vi "scan RP100 voltage.vi"(7 "data":refnum<queue>, 8 "error in (no error)":errorcluster, 11 "config in":T8={"initialize"=enum."SR830", "6221"={"6221 Resource"="GPIB1::10::INSTR", "Delta status"=FALSE, "电流|RMS(A)"=0.0}, "SR830+6221"={"source"=0, "Current(A)"=0.0, "阻抗(Ohm)"=0.0, "SR830 1"=FALSE, "SR830 2"=FALSE, "SR830 3"=FALSE, "SR830 4"=FALSE, "VISA 1"="GPIB1::1::INSTR", "VISA 2"="GPIB1::2::INSTR", "VISA 3"="GPIB1::3::INSTR", "VISA 4"="GPIB1::4::INSTR", "Reserve 1"=-1, "Reserve 2"=-1, "Reserve 3"=-1, "Reserve 4"=-1, "Sensitivity 1"=-1, "Sensitivity 2"=0, "Sensitivity 3"=-1, "Sensitivity 4"=-1, "量程入 1"=0, "量程入 2"=0, "量程入 3"=0, "量程入 4"=0}, "2400"={"2400"=FALSE, "VISA"="GPIB0::9::INSTR", "Output Level (0)"=1e-05, "Compliance  Level (0.1)"=10.0, "2400ch\n\n2400ch"=[]}, "ch"={"ch"=[], "current"=[], "change?"=[], "holding current\nwhen change ch?"=TRUE}, "Instrument"={"limit"={"Field limit"=0.0, "Field rate limit"=0.0, "Temp limit"=0.0, "Temp low limit"=0.0, "Temp rate limit "=0.0}, "genarl"={"行数"=refnum, "编辑列表框？"=refnum, "列表框"=refnum, "camg 振荡状态"=refnum, "Aborting"=refnum, "数据文件"=refnum, "warning"=refnum, "vi路径"="", "Instrument Type"=enum."PPMS"}, "cmag"={"TM620"="COM3", "M24C Resource"="GPIB0::1::INSTR", "4G supply"="GPIB0::13::INSTR", "Temp Status 24C"=refnum, "Temp"=refnum, "9T信号"=refnum, "4g supply status"=refnum, "in-plane"="", "out-plane"="", "in-plane signal"=FALSE, "out-plane signal"=FALSE, "in plane 信号"=refnum, "pzt volt"=refnum, "camg Rate"=refnum}, "lengtou2"={"750 visa"="", "750 rotate"="", "semaphore 340"=refnum, "semaphore 750"=refnum, "750 field status"=refnum, "Input (0:A) 340"=0, "340 Resource"="GPIB0::14::INSTR", "340 Status"=refnum, "Input (0:B) 340"=0, "Loop (0: 1)"=1, "Loop (1: 1)"=0, "TCP master instance"=refnum}, "lengtou"={"TCP master instance"=refnum, "335 Status"=refnum, "335 Resource "="GPIB0::24::INSTR", "Input (0:A) 335"=0, "Input (0:B) 335"=1, "Heater Output (1:1) 335"=1, "semaphore 335"=refnum}, "325 for test"={"quantum design"=refnum, "semaphore 325"=refnum, "325 Resource "="GPIB0::13::INSTR", "Input (0:A) 325"=0, "Heater Output (1:1) 325"=1, "325 Status"=refnum}}, "Aborting"=refnum, "数据文件"=refnum, "warning"=refnum, "2614B"={"2614B chA"=FALSE, "2614B chB"=FALSE, "VISA"="GPIB1::5::INSTR"}, "33522b"={"33522b resource name"="GPIB0::16::INSTR", "零电压"=0.0, "最大电压"=150.0, "间隔"=3.0, "最小电压"=-50.0, "开始扫温？"=FALSE, "loop"=3}, "gating type"=enum."2614(daul)", "RP100"={"RP100 VISA"="", "Slew"=0.0, "Voltage1"=0.0, "Reset?"=FALSE, "Voltage 2"=0.0, "interval"=0.0, "scan temp?"=FALSE}, "E4980AL"={"E4980AL VISA"="", "Function (0: Cp-D)"=0, "Signal Frequency (1000 Hz)"=1000.0}} {"E4980AL"."Function (0: Cp-D)" items=["Cp-D", "Cp-Q", "Cp-G", "Cp-Rp", "Cs-D", "Cs-Q", "Cs-Rs", "Lp-D", "Lp-Q", "Lp-G", "Lp-Rp", "Lp-Rdc", "Ls-D", "Ls-Q", "Ls-Rs", "Ls-Rdc", "R-X", "Z-thd", "Z-thr", "G-B", "Y-thd", "Y-thr", "Vdc-Idc"]; "33522b"."loop" items=["0", "1", "2", "3"]; "Instrument"."325 for test"."Heater Output (1:1) 325" items=["1"=1, "2"=2]; "Instrument"."325 for test"."Input (0:A) 325" items=["A", "B"]; "Instrument"."lengtou"."Heater Output (1:1) 335" items=["1"=1, "2"=2]; "Instrument"."lengtou"."Input (0:B) 335" items=["A", "B"]; "Instrument"."lengtou"."Input (0:A) 335" items=["A", "B"]; "Instrument"."lengtou2"."Loop (1: 1)" items=["1", "2"]; "Instrument"."lengtou2"."Loop (0: 1)" items=["1", "2"]; "Instrument"."lengtou2"."Input (0:B) 340" items=["A", "B", "C", "D"]; "Instrument"."lengtou2"."Input (0:A) 340" items=["A", "B", "C", "D"]; "SR830+6221"."Sensitivity 4" items=["Auto Gain"=-1, "2 nV/fA"=0, "5 nV/fA"=1, "10 nV/fA"=2, "20 nV/fA"=3, "50 nV/fA"=4, "100 nV/fA"=5, "200 nV/fA"=6, "500 nV/fA"=7, "1 uV/pA"=8, "2 uV/pA"=9, "5 uV/pA"=10, "10 uV/pA"=11, "20 uV/pA"=12, "50 uV/pA"=13, "100 uV/pA"=14, "200 uV/pA"=15, "500 uV/pA"=16, "1 mV/nA"=17, "2 mV/nA"=18, "5 mV/nA"=19, "10 mV/nA"=20, "20 mV/nA"=21, "50 mV/nA"=22, "100 mV/nA"=23, "200 mV/nA"=24, "500 mV/mA"=25, "1 V/uA"=26]; "SR830+6221"."Sensitivity 3" items=["Auto Gain"=-1, "2 nV/fA"=0, "5 nV/fA"=1, "10 nV/fA"=2, "20 nV/fA"=3, "50 nV/fA"=4, "100 nV/fA"=5, "200 nV/fA"=6, "500 nV/fA"=7, "1 uV/pA"=8, "2 uV/pA"=9, "5 uV/pA"=10, "10 uV/pA"=11, "20 uV/pA"=12, "50 uV/pA"=13, "100 uV/pA"=14, "200 uV/pA"=15, "500 uV/pA"=16, "1 mV/nA"=17, "2 mV/nA"=18, "5 mV/nA"=19, "10 mV/nA"=20, "20 mV/nA"=21, "50 mV/nA"=22, "100 mV/nA"=23, "200 mV/nA"=24, "500 mV/mA"=25, "1 V/uA"=26]; "SR830+6221"."Sensitivity 1" items=["Auto Gain"=-1, "2 nV/fA"=0, "5 nV/fA"=1, "10 nV/fA"=2, "20 nV/fA"=3, "50 nV/fA"=4, "100 nV/fA"=5, "200 nV/fA"=6, "500 nV/fA"=7, "1 uV/pA"=8, "2 uV/pA"=9, "5 uV/pA"=10, "10 uV/pA"=11, "20 uV/pA"=12, "50 uV/pA"=13, "100 uV/pA"=14, "200 uV/pA"=15, "500 uV/pA"=16, "1 mV/nA"=17, "2 mV/nA"=18, "5 mV/nA"=19, "10 mV/nA"=20, "20 mV/nA"=21, "50 mV/nA"=22, "100 mV/nA"=23, "200 mV/nA"=24, "500 mV/mA"=25, "1 V/uA"=26]; "SR830+6221"."Sensitivity 2" items=["Auto Gain"=-1, "2 nV/fA"=0, "5 nV/fA"=1, "10 nV/fA"=2, "20 nV/fA"=3, "50 nV/fA"=4, "100 nV/fA"=5, "200 nV/fA"=6, "500 nV/fA"=7, "1 uV/pA"=8, "2 uV/pA"=9, "5 uV/pA"=10, "10 uV/pA"=11, "20 uV/pA"=12, "50 uV/pA"=13, "100 uV/pA"=14, "200 uV/pA"=15, "500 uV/pA"=16, "1 mV/nA"=17, "2 mV/nA"=18, "5 mV/nA"=19, "10 mV/nA"=20, "20 mV/nA"=21, "50 mV/nA"=22, "100 mV/nA"=23, "200 mV/nA"=24, "500 mV/mA"=25, "1 V/uA"=26]; "SR830+6221"."Reserve 4" items=["Auto Reserve"=-1, "High Reserve"=0, "Normal"=1, "Low Noise"=2]; "SR830+6221"."Reserve 3" items=["Auto Reserve"=-1, "High Reserve"=0, "Normal"=1, "Low Noise"=2]; "SR830+6221"."Reserve 2" items=["Auto Reserve"=-1, "High Reserve"=0, "Normal"=1, "Low Noise"=2]; "SR830+6221"."Reserve 1" items=["Auto Reserve"=-1, "High Reserve"=0, "Normal"=1, "Low Noise"=2]; "SR830+6221"."source" items=["SR830 1", "SR830 2", "SR830 3", "SR830 4"]}) -> (0 "error out":errorcluster, 3 "config in 2":T1={"initialize"=enum."SR830", "6221"={"6221 Resource"="GPIB0::24::INSTR", "Delta status"=FALSE, "电流|RMS(A)"=0.0}, "SR830+6221"={"source"=0, "Current(A)"=0.0, "阻抗(Ohm)"=0.0, "SR830 1"=FALSE, "SR830 2"=FALSE, "SR830 3"=FALSE, "SR830 4"=FALSE, "VISA 1"="", "VISA 2"="", "VISA 3"="", "VISA 4"="", "Reserve 1"=-1, "Reserve 2"=-1, "Reserve 3"=-1, "Reserve 4"=-1, "Sensitivity 1"=-1, "Sensitivity 2"=-1, "Sensitivity 3"=-1, "Sensitivity 4"=-1, "量程入 1"=0, "量程入 2"=0, "量程入 3"=0, "量程入 4"=0}, "2400"={"2400"=FALSE, "VISA"="GPIB0::9::INSTR", "Output Level (0)"=1e-05, "Compliance  Level (0.1)"=10.0, "ch"=[]}, "ch"={"ch"=[], "current"=[], "change?"=[], "holding current\nwhen change ch?"=FALSE, "current offset"=[]}, "Instrument"={"limit"={"Field limit"=0.0, "Field rate limit"=0.0, "Temp limit"=0.0, "Temp low limit"=0.0, "Temp rate limit "=0.0}, "genarl"={"行数"=refnum, "编辑列表框？"=refnum, "列表框"=refnum, "camg 振荡状态"=refnum, "Aborting"=refnum, "数据文件"=refnum, "warning"=refnum, "vi路径"="", "Instrument Type"=enum."SVSM"}, "cmag"={"TM620"="GPIB0::24::INSTR", "M24C Resource"="GPIB0::24::INSTR", "4G supply"="GPIB0::24::INSTR", "Temp Status 24C"=refnum, "Temp"=refnum, "9T信号"=refnum, "4g supply status"=refnum, "in-plane"="", "out-plane"="", "in-plane signal"=TRUE, "out-plane signal"=FALSE, "in plane 信号"=refnum, "pzt volt"=refnum, "camg Rate"=refnum}, "lengtou2"={"750 visa"="", "750 rotate"="", "semaphore 340"=refnum, "semaphore 750"=refnum, "750 field status"=refnum, "Input (0:A) 340"=1, "340 Resource"="GPIB0::14::INSTR", "340 Status"=refnum, "Input (0:B) 340"=0, "Loop (0: 1)"=1, "Loop (1: 1)"=0, "TCP master instance"=refnum}, "lengtou"={"TCP master instance"=refnum, "335 Status"=refnum, "335 Resource "="GPIB0::24::INSTR", "Input (0:A) 335"=0, "Input (0:B) 335"=0, "Heater Output (1:1) 335"=0, "semaphore 335"=refnum}, "325 for test"={"quantum design"=refnum, "semaphore 325"=refnum, "325 Resource "="GPIB0::13::INSTR", "Input (0:A) 325"=1000, "Heater Output (1:1) 325"=1, "325 Status"=refnum}}, "2614B"={"2614B chA"=FALSE, "2614B chB"=FALSE, "VISA"=""}, "33522b"={"33522b resource name"="GPIB0::16::INSTR", "零电压"=0.0, "最大电压"=148.0, "间隔"=4.0, "最小电压"=-48.0, "loop"=3.0, "压电陶瓷电压(Vpp)"=0.0}, "gating type"=enum."2614(daul)", "层数"=0, "行数"=0, "是否处理"=[], "current 2"=[], "StrainCell"={"RP100 resource name"="GPIB0::16::INSTR", "E4980 resource name"="GPIB0::16::INSTR", "RP100 Reset ?(True)"=TRUE, "Voltage1(V)"=0.0, "Voltage2(V)"=0.0, "interval"=4.0, "slew(V/s)"=1.0}} {"Instrument"."325 for test"."Heater Output (1:1) 325" items=["1"=1, "2"=2]; "Instrument"."325 for test"."Input (0:A) 325" items=["A", "B"]; "Instrument"."lengtou"."Heater Output (1:1) 335" items=["1"=1, "2"=2]; "Instrument"."lengtou"."Input (0:B) 335" items=["A", "B"]; "Instrument"."lengtou"."Input (0:A) 335" items=["A", "B"]; "Instrument"."lengtou2"."Loop (1: 1)" items=["1", "2"]; "Instrument"."lengtou2"."Loop (0: 1)" items=["1", "2"]; "Instrument"."lengtou2"."Input (0:B) 340" items=["A", "B", "C", "D"]; "Instrument"."lengtou2"."Input (0:A) 340" items=["A", "B", "C", "D"]; "SR830+6221"."Sensitivity 4" items=["Auto Gain"=-1, "2 nV/fA"=0, "5 nV/fA"=1, "10 nV/fA"=2, "20 nV/fA"=3, "50 nV/fA"=4, "100 nV/fA"=5, "200 nV/fA"=6, "500 nV/fA"=7, "1 uV/pA"=8, "2 uV/pA"=9, "5 uV/pA"=10, "10 uV/pA"=11, "20 uV/pA"=12, "50 uV/pA"=13, "100 uV/pA"=14, "200 uV/pA"=15, "500 uV/pA"=16, "1 mV/nA"=17, "2 mV/nA"=18, "5 mV/nA"=19, "10 mV/nA"=20, "20 mV/nA"=21, "50 mV/nA"=22, "100 mV/nA"=23, "200 mV/nA"=24, "500 mV/mA"=25, "1 V/uA"=26]; "SR830+6221"."Sensitivity 3" items=["Auto Gain"=-1, "2 nV/fA"=0, "5 nV/fA"=1, "10 nV/fA"=2, "20 nV/fA"=3, "50 nV/fA"=4, "100 nV/fA"=5, "200 nV/fA"=6, "500 nV/fA"=7, "1 uV/pA"=8, "2 uV/pA"=9, "5 uV/pA"=10, "10 uV/pA"=11, "20 uV/pA"=12, "50 uV/pA"=13, "100 uV/pA"=14, "200 uV/pA"=15, "500 uV/pA"=16, "1 mV/nA"=17, "2 mV/nA"=18, "5 mV/nA"=19, "10 mV/nA"=20, "20 mV/nA"=21, "50 mV/nA"=22, "100 mV/nA"=23, "200 mV/nA"=24, "500 mV/mA"=25, "1 V/uA"=26]; "SR830+6221"."Sensitivity 1" items=["Auto Gain"=-1, "2 nV/fA"=0, "5 nV/fA"=1, "10 nV/fA"=2, "20 nV/fA"=3, "50 nV/fA"=4, "100 nV/fA"=5, "200 nV/fA"=6, "500 nV/fA"=7, "1 uV/pA"=8, "2 uV/pA"=9, "5 uV/pA"=10, "10 uV/pA"=11, "20 uV/pA"=12, "50 uV/pA"=13, "100 uV/pA"=14, "200 uV/pA"=15, "500 uV/pA"=16, "1 mV/nA"=17, "2 mV/nA"=18, "5 mV/nA"=19, "10 mV/nA"=20, "20 mV/nA"=21, "50 mV/nA"=22, "100 mV/nA"=23, "200 mV/nA"=24, "500 mV/mA"=25, "1 V/uA"=26]; "SR830+6221"."Sensitivity 2" items=["Auto Gain"=-1, "2 nV/fA"=0, "5 nV/fA"=1, "10 nV/fA"=2, "20 nV/fA"=3, "50 nV/fA"=4, "100 nV/fA"=5, "200 nV/fA"=6, "500 nV/fA"=7, "1 uV/pA"=8, "2 uV/pA"=9, "5 uV/pA"=10, "10 uV/pA"=11, "20 uV/pA"=12, "50 uV/pA"=13, "100 uV/pA"=14, "200 uV/pA"=15, "500 uV/pA"=16, "1 mV/nA"=17, "2 mV/nA"=18, "5 mV/nA"=19, "10 mV/nA"=20, "20 mV/nA"=21, "50 mV/nA"=22, "100 mV/nA"=23, "200 mV/nA"=24, "500 mV/mA"=25, "1 V/uA"=26]; "SR830+6221"."Reserve 4" items=["Auto Reserve"=-1, "High Reserve"=0, "Normal"=1, "Low Noise"=2]; "SR830+6221"."Reserve 3" items=["Auto Reserve"=-1, "High Reserve"=0, "Normal"=1, "Low Noise"=2]; "SR830+6221"."Reserve 2" items=["Auto Reserve"=-1, "High Reserve"=0, "Normal"=1, "Low Noise"=2]; "SR830+6221"."Reserve 1" items=["Auto Reserve"=-1, "High Reserve"=0, "Normal"=1, "Low Noise"=2]; "SR830+6221"."source" items=["SR830 1", "SR830 2", "SR830 3", "SR830 4"]})   [LabVIEW 2019]
uses:
  lib/RP100/RP100.lvlib
  nematic/Copy of StrainCell.lvlib
  <vilib>/NI/Modbus Library/API/Master/Modbus Master.lvclass
  C:/Program Files (x86)/National Instruments/LabVIEW 2019/vi.lib/NI/Modbus Library/API/Modbus API.lvclass
  ctl/initialize.ctl
  ctl/Instrument Type.ctl
  ctl/335 state.ctl
  ctl/limit.ctl
  ctl/9T mag field stauts.ctl
  ctl/Instrument.ctl
  ctl/warning.ctl
  ctl/Gating type.ctl
  ctl/config.ctl
  C:/Users/fuyang/Desktop/postdoctor/labview/labview-measure/lib/QDInstrument.dll
  lib/QDInstrument.dll
  jigui/Desktop/labview-measure-master240417/labview-measure-master-230926/configs/Control 1.ctl
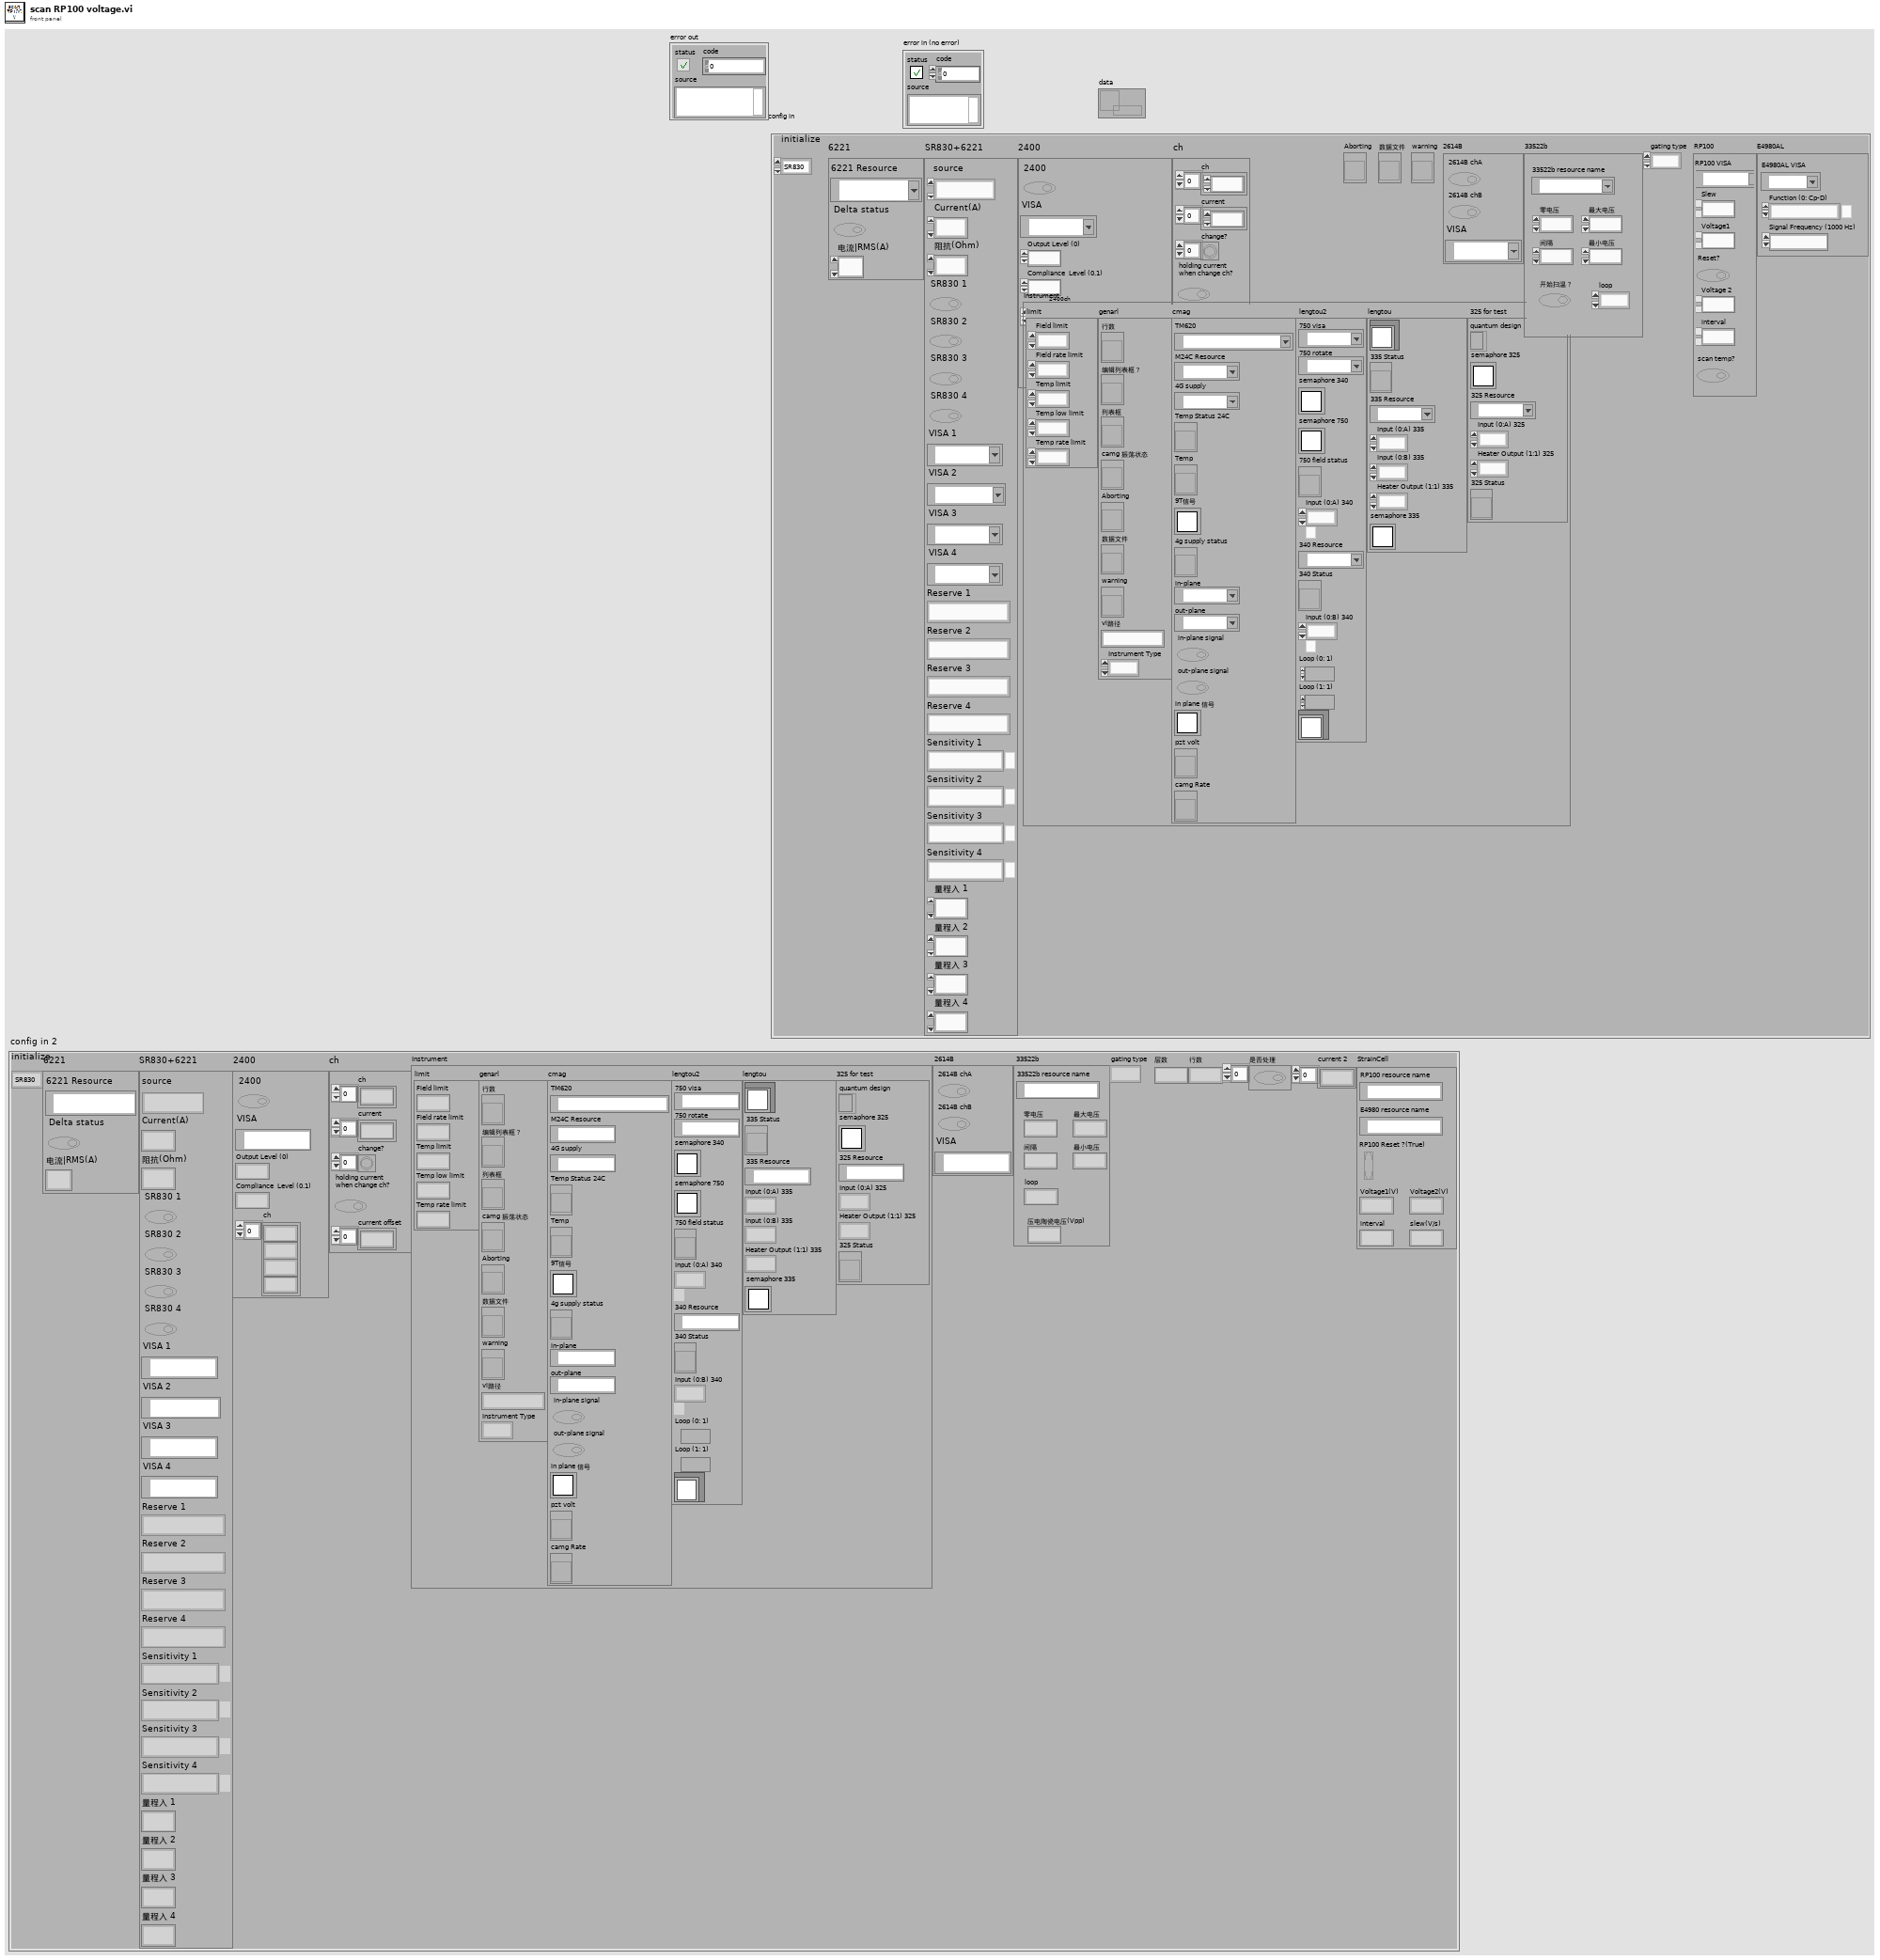
[diagram p1: front panel]
types:
  T1 = typedef "config.ctl" = cluster{"initialize":T2, "6221":cluster{"6221 Resource":refnum<visa-resource-name>, "Delta status":bool, "电流|RMS(A)":dbl}, "SR830+6221":cluster{"source":u16, "Current(A)":dbl, "阻抗(Ohm)":dbl, "SR830 1":bool, "SR830 2":bool, "SR830 3":bool, "SR830 4":bool, "VISA 1":refnum<visa-resource-name>, "VISA 2":refnum<visa-resource-name>, "VISA 3":refnum<visa-resource-name>, "VISA 4":refnum<visa-resource-name>, "Reserve 1":i16, "Reserve 2":i16, "Reserve 3":i16, "Reserve 4":i16, "Sensitivity 1":i16, "Sensitivity 2":i16, "Sensitivity 3":i16, "Sensitivity 4":i16, "量程入 1":i32, "量程入 2":i32, "量程入 3":i32, "量程入 4":i32}, "2400":cluster{"2400":bool, "VISA":refnum<visa-resource-name>, "Output Level (0)":dbl, "Compliance  Level (0.1)":dbl, "ch":i32[]}, "ch":cluster{"ch":i32[], "current":dbl[], "change?":bool[], "holding current\nwhen change ch?":bool, "current offset":dbl[]}, "Instrument":T3, "2614B":cluster{"2614B chA":bool, "2614B chB":bool, "VISA":refnum<visa-resource-name>}, "33522b":cluster{"33522b resource name":refnum<visa-resource-name>, "零电压":dbl, "最大电压":dbl, "间隔":dbl, "最小电压":dbl, "loop":dbl, "压电陶瓷电压(Vpp)":dbl}, "gating type":T7, "层数":i32, "行数":i32, "是否处理":bool[], "current 2":dbl[], "StrainCell":cluster{"RP100 resource name":refnum<visa-resource-name>, "E4980 resource name":refnum<visa-resource-name>, "RP100 Reset ?(True)":bool, "Voltage1(V)":dbl, "Voltage2(V)":dbl, "interval":dbl, "slew(V/s)":dbl}}
  T2 = typedef "initialize.ctl" = enum16{"SR830", "keithley6221-SR830", "Delta", "Delta-tunnelling", "keithley6221-2182-DC", "PZT", "StrainCell", "4200"}
  T3 = typedef "Instrument.ctl" = cluster{"limit":T4, "genarl":cluster{"行数":refnum<vi>, "编辑列表框？":refnum<vi>, "列表框":refnum<vi>, "camg 振荡状态":refnum<vi>, "Aborting":refnum<vi>, "数据文件":refnum<vi>, "warning":refnum<vi>, "vi路径":string, "Instrument Type":T5}, "cmag":cluster{"TM620":refnum<visa-resource-name>, "M24C Resource":refnum<visa-resource-name>, "4G supply":refnum<visa-resource-name>, "Temp Status 24C":refnum<vi>, "Temp":refnum<vi>, "9T信号":T6, "4g supply status":refnum<vi>, "in-plane":refnum<visa-resource-name>, "out-plane":refnum<visa-resource-name>, "in-plane signal":bool, "out-plane signal":bool, "in plane 信号":T6, "pzt volt":refnum<vi>, "camg Rate":refnum<vi>}, "lengtou2":cluster{"750 visa":refnum<visa-resource-name>, "750 rotate":refnum<visa-resource-name>, "semaphore 340":T6, "semaphore 750":T6, "750 field status":refnum<vi>, "Input (0:A) 340":u16, "340 Resource":refnum<visa-resource-name>, "340 Status":refnum<vi>, "Input (0:B) 340":u16, "Loop (0: 1)":u16, "Loop (1: 1)":u16, "TCP master instance":refnum<class "Modbus Master.lvclass">}, "lengtou":cluster{"TCP master instance":refnum<class "Modbus Master.lvclass">, "335 Status":refnum<vi>, "335 Resource ":refnum<visa-resource-name>, "Input (0:A) 335":u16, "Input (0:B) 335":u16, "Heater Output (1:1) 335":u16, "semaphore 335":T6}, "325 for test":cluster{"quantum design":refnum<k24>, "semaphore 325":T6, "325 Resource ":refnum<visa-resource-name>, "Input (0:A) 325":u16, "Heater Output (1:1) 325":u16, "325 Status":refnum<vi>}}
  T4 = typedef "limit.ctl" = cluster{"Field limit":dbl, "Field rate limit":dbl, "Temp limit":dbl, "Temp low limit":dbl, "Temp rate limit ":dbl}
  T5 = typedef "Instrument Type.ctl" = enum16{"PPMS", "VersaLab", "DynaCool", "SVSM", "PPMS-Rotate", "Lakeshore335", "2T cmag", "9T mag old", "9T cmag", "9T cmag DAC", "9T cmag rotate", "test"}
  T6 = typedef "Semaphore RefNum" = refnum<k1>
  T7 = typedef "Gating type.ctl" = enum32{"null", "2614(daul)", "2400", "6517B"}
  T8 = typedef "config.ctl" = cluster{"initialize":T2, "6221":cluster{"6221 Resource":refnum<visa-resource-name>, "Delta status":bool, "电流|RMS(A)":dbl}, "SR830+6221":cluster{"source":u16, "Current(A)":dbl, "阻抗(Ohm)":dbl, "SR830 1":bool, "SR830 2":bool, "SR830 3":bool, "SR830 4":bool, "VISA 1":refnum<visa-resource-name>, "VISA 2":refnum<visa-resource-name>, "VISA 3":refnum<visa-resource-name>, "VISA 4":refnum<visa-resource-name>, "Reserve 1":i16, "Reserve 2":i16, "Reserve 3":i16, "Reserve 4":i16, "Sensitivity 1":i16, "Sensitivity 2":i16, "Sensitivity 3":i16, "Sensitivity 4":i16, "量程入 1":i32, "量程入 2":i32, "量程入 3":i32, "量程入 4":i32}, "2400":cluster{"2400":bool, "VISA":refnum<visa-resource-name>, "Output Level (0)":dbl, "Compliance  Level (0.1)":dbl, "2400ch\n\n2400ch":T9[]}, "ch":cluster{"ch":i32[], "current":dbl[], "change?":bool[], "holding current\nwhen change ch?":bool}, "Instrument":T3, "Aborting":refnum<vi>, "数据文件":refnum<vi>, "warning":refnum<vi>, "2614B":cluster{"2614B chA":bool, "2614B chB":bool, "VISA":refnum<visa-resource-name>}, "33522b":cluster{"33522b resource name":refnum<visa-resource-name>, "零电压":dbl, "最大电压":dbl, "间隔":dbl, "最小电压":dbl, "开始扫温？":bool, "loop":u16}, "gating type":T7, "RP100":cluster{"RP100 VISA":refnum<visa-resource-name>, "Slew":dbl, "Voltage1":dbl, "Reset?":bool, "Voltage 2":dbl, "interval":dbl, "scan temp?":bool}, "E4980AL":cluster{"E4980AL VISA":refnum<visa-resource-name>, "Function (0: Cp-D)":u16, "Signal Frequency (1000 Hz)":dbl}}
  T9 = typedef "Control 1.ctl" = i32
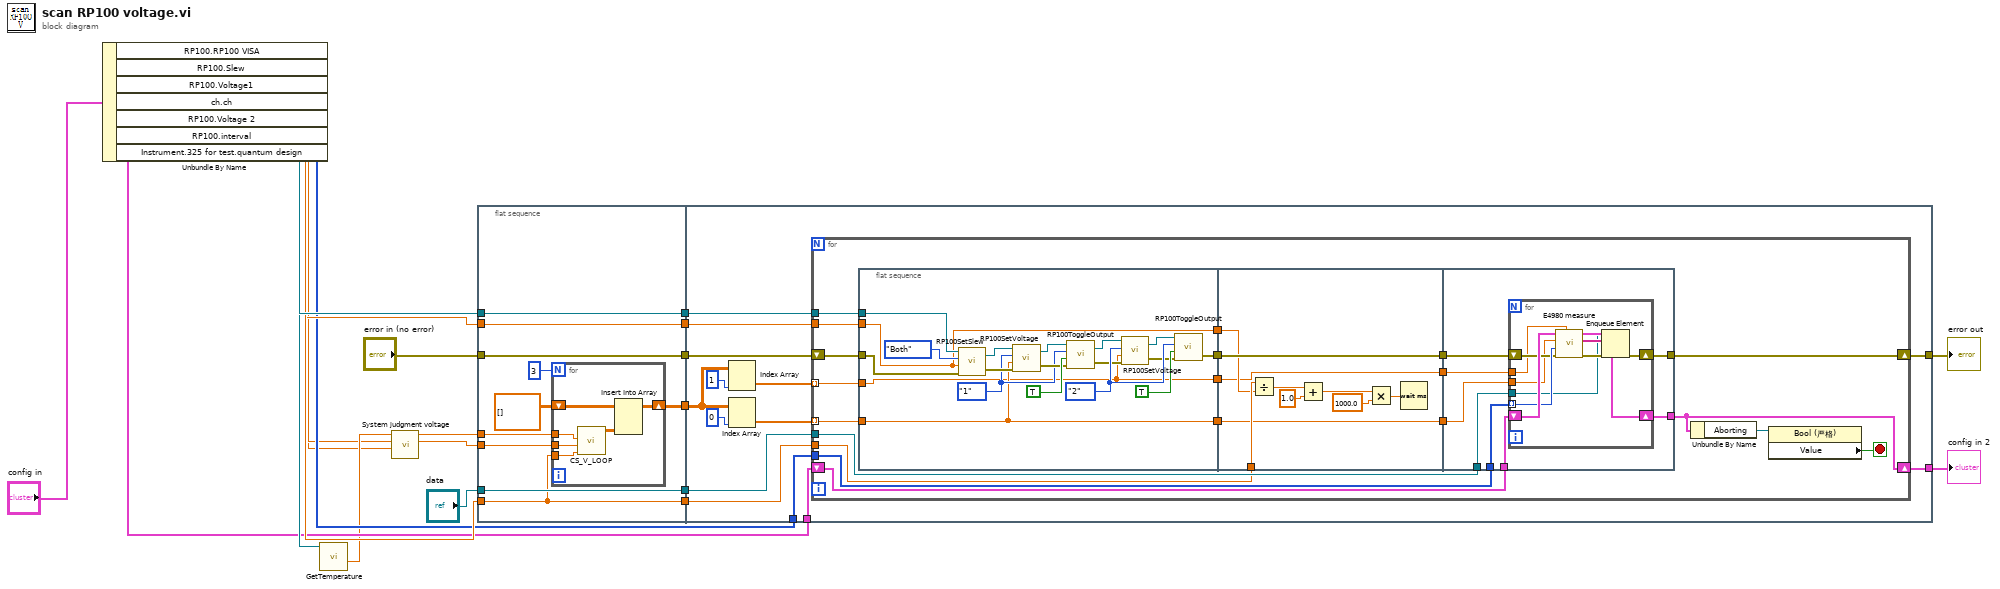
[diagram p0: block diagram]
diagram:
  n1 = Unbundle By Name("config in") -> ("RP100.RP100 VISA"=w19:refnum<visa-resource-name>, "RP100.Slew"=w12:dbl, "RP100.Voltage1"=w4:dbl, "ch.ch"=w11:i32[], "RP100.Voltage 2"=w3:dbl, "RP100.interval"=w13:dbl, "Instrument.325 for test.quantum design"=w7:refnum<k24>)
  n2 = call "GetTemperature.vi"("Instrument Ref In"=w7) -> ("Temperature"=w5:dbl)  [unwired: 4 in, 4 out]
  n3 = call "System judgment voltage.vi"(9:w3, 10:w4, "Temperature"=w5) -> ("Voltage 2"=w1:dbl, "Voltage 1"=w2:dbl)  [unwired: 7 in]
  n4 = flat-sequence {
    tunnel: "data" -> [w29]
    tunnel: w2 -> [w28]
    tunnel: w12 -> [w26]
    tunnel: w19 -> [w30]
    tunnel: "error in (no error)" -> [w31]
    tunnel: [w31] -> w18
    tunnel: [w30] -> w17
    tunnel: [w26] -> w16
    tunnel: [w24] -> w15
    tunnel: [w29] -> w14
    tunnel: w1 -> [w27]
    tunnel: w13 -> [w23]
    tunnel: [w23] -> w8
    tunnel: w18 -> [w51]
    tunnel: w17 -> [w48]
    tunnel: w16 -> [w50]
    tunnel: w15 -> [w39]
    tunnel: w14 -> [w49]
    tunnel: w11 -> [w47]
    tunnel: "config in" -> [w46]
    tunnel: [w45] -> w10
    tunnel: [w44] -> w9
    tunnel: w8 -> [w43]
    frame #0 {
      n5 = for {
        N: 3 -> [_]
        tunnel: w28 -> [w37]
        tunnel: w27 -> [w36]
        tunnel: w23 -> [w35]
        shift-right: [w34] -> w24
        shift-left: dbl[][] [] -> [w33]
        n6 = call "CS_V_LOOP.vi"("间隔"=w35, "最小电压"=w36, "最大电压"=w37) -> ("output array"=w32:dbl[][])  [unwired: 8 in]
        n7 = Insert Into Array(array=w33, new element=w32) -> (w34:dbl[][])  [unwired: 2 in]
      }
    }
    frame #1 {
      n8 = Index Array(array=w39, index (col)=1 ("disabled index (col)")) -> (element=w38:dbl[])  [unwired: 1 in]
      n9 = Index Array(array=w39, index (col)=0 ("disabled index (col)")) -> (element=w41:dbl[])  [unwired: 1 in]
      n10 = for {
        tunnel: w50 -> [w70]
        tunnel: w41 -> [w69] mode=indexing
        tunnel: w49 -> [w65]
        tunnel: w48 -> [w68]
        tunnel: w47 -> [w55]
        shift-right: [w63] -> w45
        shift-left: w51 -> [w71]
        shift-right: [w59] -> w44
        shift-left: w46 -> [w64]
        tunnel: w43 -> [w62]
        tunnel: w38 -> [w54] mode=indexing
        stop <- w58 stop-if-true
        n11 = flat-sequence {
          tunnel: w71 -> [w88]
          tunnel: w70 -> [w82]
          tunnel: w69 -> [w73]
          tunnel: w68 -> [w84]
          tunnel: [w74] -> w67
          tunnel: [w82] -> w61
          tunnel: [w73] -> w57
          tunnel: w54 -> [w72]
          tunnel: [w72] -> w53
          tunnel: w67 -> [w100]
          tunnel: [w100] -> w66
          tunnel: w62 -> [w99]
          tunnel: w61 -> [w98]
          tunnel: w57 -> [w96]
          tunnel: [w96] -> w56
          tunnel: w53 -> [w91]
          tunnel: [w91] -> w52
          tunnel: w66 -> [w106]
          tunnel: w55 -> [w108]
          tunnel: w65 -> [w107]
          tunnel: w64 -> [w105]
          tunnel: [w104] -> w63
          tunnel: [w103] -> w59
          tunnel: w56 -> [w102]
          tunnel: w52 -> [w101]
          frame #0 {
            w78 = enum16{"1", "2", "Both"}."2" ("Source")
            w79 = enum16{"1", "2", "Both"}."1" ("Source")
            n12 = call "RP100SetSlew.vi"("error in (no error)"=w88, "Slew"=w82, "Source"=enum16{"1", "2", "Both"}."Both", "VISA resource name"=w84) -> ("error out"=w89:errorcluster, "VISA resource name out"=w90:refnum<visa-resource-name>)
            n13 = call "RP100SetVoltage.vi"("error in (no error)"=w89, "Voltage"=w73, "Source"=w79, "VISA resource name"=w90) -> ("error out"=w85:errorcluster, "VISA resource name out"=w87:refnum<visa-resource-name>)
            n14 = call "RP100ToggleOutput.vi"("error in (no error)"=w85, "Enable?"=TRUE, "Source"=w79, "VISA resource name"=w87) -> ("error out"=w76:errorcluster, "VISA resource name out"=w81:refnum<visa-resource-name>)
            n15 = call "RP100SetVoltage.vi"("error in (no error)"=w76, "Voltage"=w72, "Source"=w78, "VISA resource name"=w81) -> ("error out"=w75:errorcluster, "VISA resource name out"=w80:refnum<visa-resource-name>)
            n16 = call "RP100ToggleOutput.vi"("error in (no error)"=w75, "Enable?"=TRUE, "Source"=w78, "VISA resource name"=w80) -> ("error out"=w74:errorcluster)  [unwired: 1 out]
          }
          frame #1 {
            n17 = Divide(x=w99, y=w98) -> (x/y=w95:dbl)
            n18 = Add(x=w95, y=1.0) -> (x+y=w94:dbl)
            n19 = Multiply(x=w94, y=1000.0) -> (x*y=w93:dbl)
            n20 = Wait (ms)(milliseconds to wait=w93) -> ()  [unwired: 1 out]
          }
          frame #2 {
            n21 = for {
              tunnel: w108 -> [w117] mode=indexing
              tunnel: w107 -> [w111]
              shift-right: [w113] -> w103
              shift-left: w105 -> [w118]
              shift-right: [w114] -> w104
              shift-left: w106 -> [w116]
              tunnel: w102 -> [w110]
              tunnel: w101 -> [w109]
              n22 = call "E4980 measure.vi"("set V2"=w109, "错误输入（无错误）"=w116, "ch"=w117, "set V1"=w110, "config1"=w118) -> ("错误输出"=w115:errorcluster, "添加的数组"=w112:string[], "输出簇"=w113:T1)  [unwired: 4 in]
              n23 = Enqueue Element(queue=w111, element=w112, error in (no error)=w115) -> (error out=w114:errorcluster)  [unwired: 1 in, 2 out]
            }
          }
        }
        n24 = Unbundle By Name(w59) -> ("Aborting"=w60:refnum<vi>)
        n25 = property class="Bool (严格)"(reference=w60) -> ("Value"=w58:bool)  [unwired: 1 in, 2 out]
      }
    }
  }
  "error out" <- w10
  "config in 2" <- w9
